vi "Save keep old plots.vi"(8 "error in (no error)":errorcluster, 11 "MagLabGraph in":refnum<class "XY Plot.lvclass">) -> (0 "error out":errorcluster, 2 "Value":bool, 3 "MagLabGraph out":refnum<class "XY Plot.lvclass">)   [LabVIEW 2015, in "XY Plot.lvclass"]
uses:
  XY Plot.lvclass
  XY Plot.lvclass/XY Plot.ctl
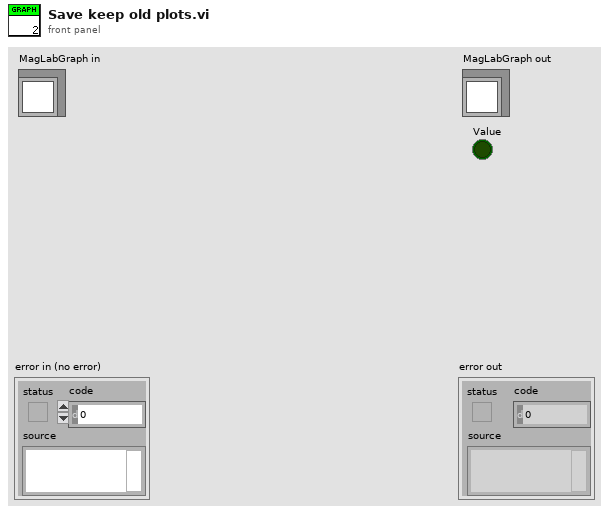
[diagram p1: front panel]
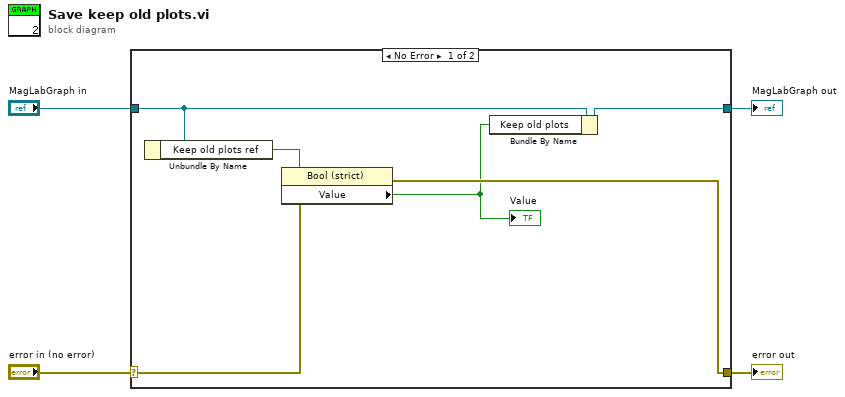
[diagram p0: block diagram]
diagram:
  n1 = case shown="No Error" "error in (no error)" {
    selector: "error in (no error)" -> [w9 w12]
    tunnel: [w8 w12] -> w3
    tunnel: [w6 w11] -> w1
    tunnel: "MagLabGraph in" -> [w10 w11]
    frame No Error {
      n2 = Unbundle By Name(w10) -> ("Keep old plots ref"=w7:refnum<vi>)
      n3 = property class="Bool (strict)"(reference=w7, error in=w9) -> (error out=w8:errorcluster, "Value"=w5:bool)  [unwired: 1 out]
      "Value" <- w5
      n4 = Bundle By Name(cluster=w10, "Keep old plots"=w5) -> (w6:refnum<class "XY Plot.lvclass">)
    }
    frame Error {
    }
  }
  "error out" <- w3
  "MagLabGraph out" <- w1
